vi "SCT Is Variant NULL.vi"(1 "Type Descriptor":T1) -> (0 "NULL?":bool)   [LabVIEW 2016]
uses:
  <vilib>/variable/Type Descriptor.ctl
  <vilib>/variable/NI_Variable.lvlib
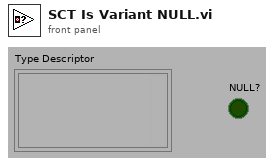
[diagram p1: front panel]
types:
  T1 = typedef "NI_Variable.lvlib/Type Descriptor.ctl" = cluster{"Variant":variant}
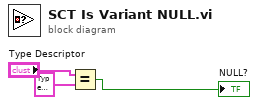
[diagram p0: block diagram]
diagram:
  n1 = Equal?(x="Type Descriptor", y=T1 {"Variant"=variant}) -> (x = y?=→"NULL?":bool)
